vi "Clean Up.vi"(8 "error in (no error)":errorcluster, 11 "Robotiq in":refnum<class "Robotiq.lvclass">) -> (0 "error out":errorcluster, 3 "Robotiq out":refnum<class "Robotiq.lvclass">)   [LabVIEW 2011, in "Robotiq.lvclass"]
uses:
  Robotiq.lvclass
  Robotiq.lvclass/Robotiq.ctl
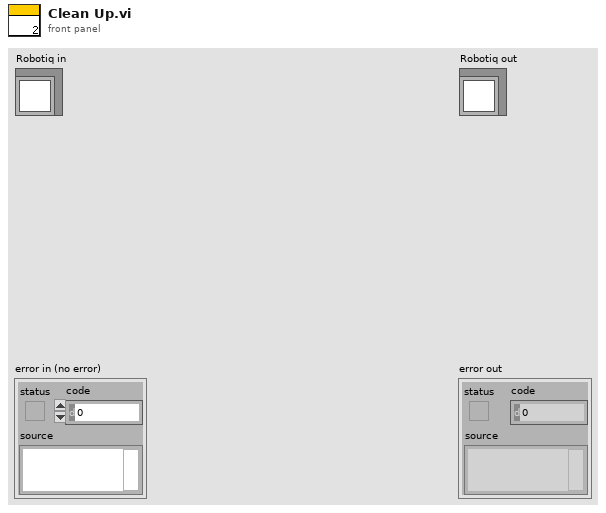
[diagram p1: front panel]
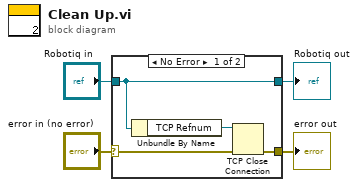
[diagram p0: block diagram]
diagram:
  n1 = case shown="No Error" "error in (no error)" {
    selector: "error in (no error)" -> [w8 w10]
    tunnel: [w7 w10] -> w3
    tunnel: [w6 w9] -> w1
    tunnel: "Robotiq in" -> [w6 w9]
    frame No Error {
      n2 = Unbundle By Name(w6) -> ("TCP Refnum"=w5:refnum<k5>)
      n3 = TCP Close Connection(connection ID=w5, error in (no error)=w8) -> (error out=w7:errorcluster)  [unwired: 1 in, 1 out]
    }
    frame Error {
    }
  }
  "error out" <- w3
  "Robotiq out" <- w1
